vi "lab2_usrp_packet_transceiver2.vi"() -> ()   [LabVIEW 2014]
uses:
  <vilib>/addons/Modulation/Digital/General/MT Generate Bits (Galois, PN Order).vi
  <vilib>/addons/Modulation/Analog/support/mod_Set Error Source.vi
  <vilib>/addons/Modulation/Digital/Support/Common/Validators/mod_Generate Bits Validate.vi
  var_stop.vi
  <vilib>/addons/Modulation/Digital/Support/Common/Validators/mod_Generate Filter Coefficients Validate.vi
  <vilib>/addons/Modulation/Digital/General/subVIs/mod_Generate Filter Coefficients.vi
  <vilib>/measure/maspectr.llb/FFT Power Spectrum and PSD for 1 Chan (CDB).vi
  <vilib>/addons/Modulation/Digital/General/MT Apply Matched Filter (Generic).vi
  <vilib>/addons/Modulation/Digital/General/MT Align to Ideal Symbols (Generic).vi
  <instrlib>/niUSRP/niUSRP Fetch Rx Data (CDB Cluster).vi
  <instrlib>/niUSRP/niUSRP Write Tx Data (CDB Cluster).vi
  <vilib>/addons/Modulation/Digital/General/subVIs/mod_Generate Bits PN Sequence.vi
  <vilib>/addons/Modulation/Digital/General/MT Apply Pulse Shaping Filter (Generic).vi
  <vilib>/addons/Modulation/niDMT.lvlib
  <vilib>/measure/NI_MAPro.lvlib
panel:
  out "ser":dbl
  out "received symbols":dbl
  out "error symbols":i32
  in  "random bits length":i32=50000
  in  "packet bits":i32[](array[numeric])
  out "RX Constellation Map (uneq)":cdb[](graph)
  in  "Transmit power (db)":dbl
  out "ber":dbl
  out "received bits":i32
  out "error bits":i32
  in  "random bits":i8[](array[numeric])
  out "found?":bool
  out "# elements in queue":i32
  out "Spectrum monitor":cluster{"f0":dbl, "df":dbl, "magnitude":dbl[]}(graph)={"f0"=-0.49993781867926873, "df"=0.00012436264146250465, "magnitude"=[]}
  out "RX Constellation Map":cdb[](graph)
  out "valid?":bool
  in  "Gray code?":bool
  in  "Modulation":enum16{"PSK", "QAM"}(ring)=enum."QAM"
  out "Rx String":string
  out "packet len":u32
  in  "Send":bool
  in  "filter length (symbols)":i32=8
  in  "filter parameter":dbl=0.5 format="%.2f"
  in  "pulse shaping filter (none)":T1(ring)=enum."Raised Cosine"
  in  "M-PSK (4)":i32=16 caption="M-ARY"
  in  "samples per symbol (16)":i32=4
  out "packet bits length":i32
  in  "number of samples":i64=40000
  out "RX coerced gain":dbl format="%#_6f"
  out "RX coerced carrier frequency":dbl=915000000.0 format="%#_6p"
  out "RX coerced IQ rate":dbl=4000000.0 format="%#_6p"
  in  "RX active antenna":string="RX2"
  in  "RX gain":dbl format="%#_6f"
  in  "RX device names":refnum<k15>="192.168.10.2"
  out "TX coerced gain":dbl format="%#_6f"
  out "TX coerced carrier frequency":dbl=915000000.0 format="%#_6p"
  out "coerced IQ rate":dbl=4000000.0 format="%#_6p"
  in  "TX device names":refnum<k15>="192.168.10.2"
  in  "TX gain":dbl format="%#_6f"
  in  "carrier frequency":dbl=915000000.0 format="%#_6p"
  in  "IQ rate":dbl=800000.0 format="%#_6p"
  in  "stop":bool
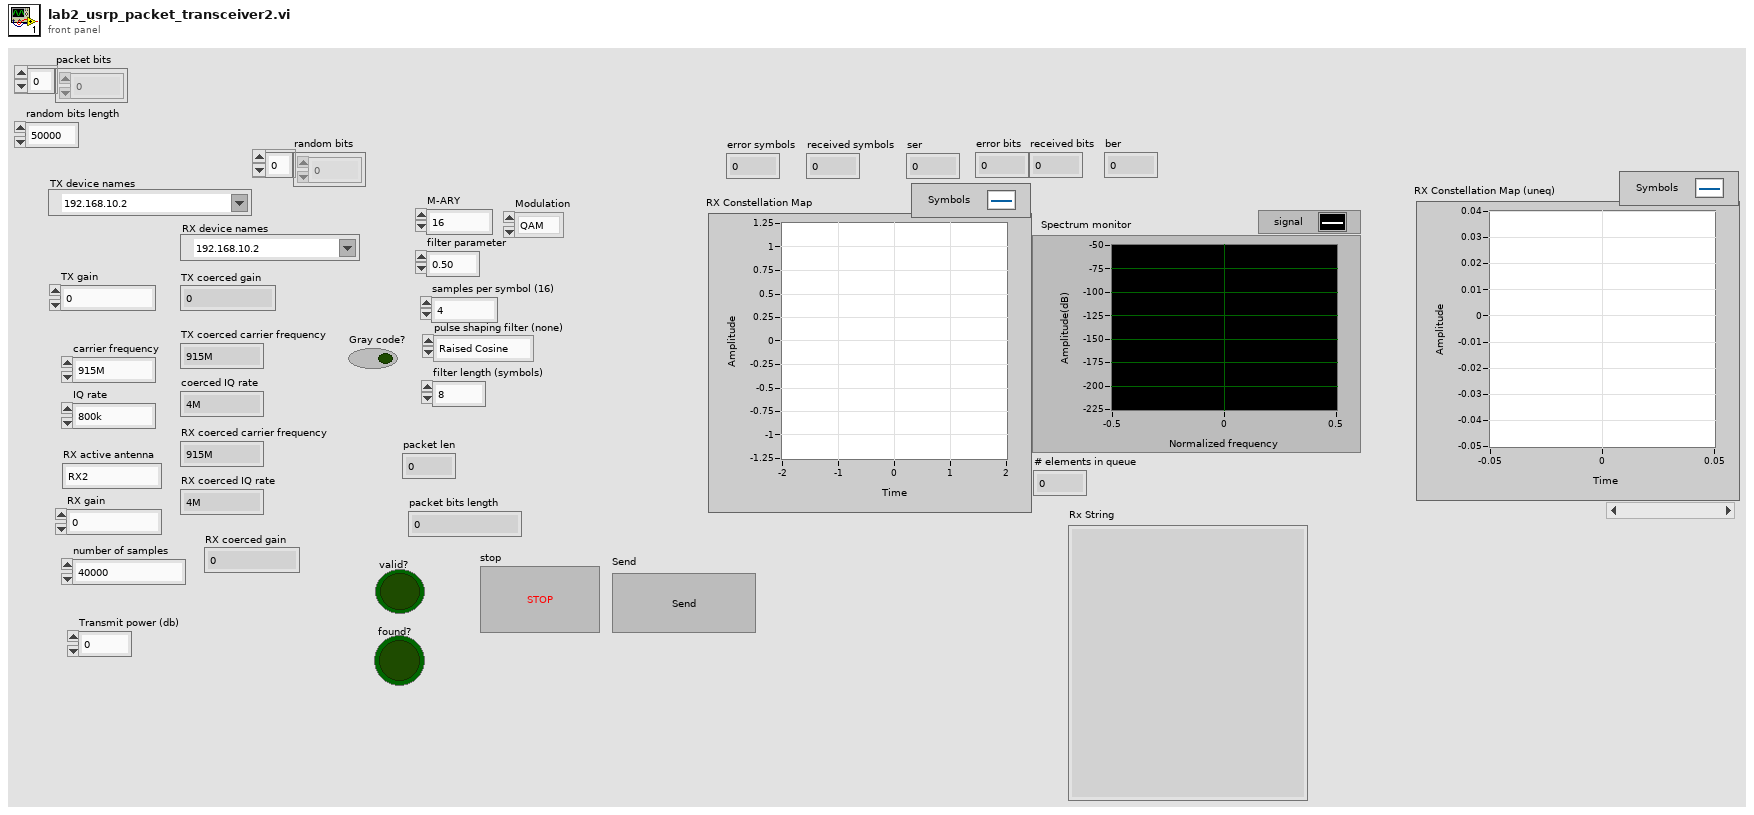
[diagram p1: front panel]
types:
  T1 = enum16{"none", "Raised Cosine", "Root Raised Cos", "Gaussian"}
  T2 = enum16{"FSK", "PSK", "QAM", "MSK", "PAM", "ASK", "CPM"}
  T3 = cluster{"samples per symbol (16)":i32, "symbol map":cdb[], "index map":u32[]}
  T4 = cluster{"samples per symbol (16)":i32, "symbol map":cdb[], i32[]}
  T5 = typedef "niAMT.lvlib/Complex Data Waveform.ctl" = cluster{"t0":dbl, "dt":dbl, "Y":cdb[]}
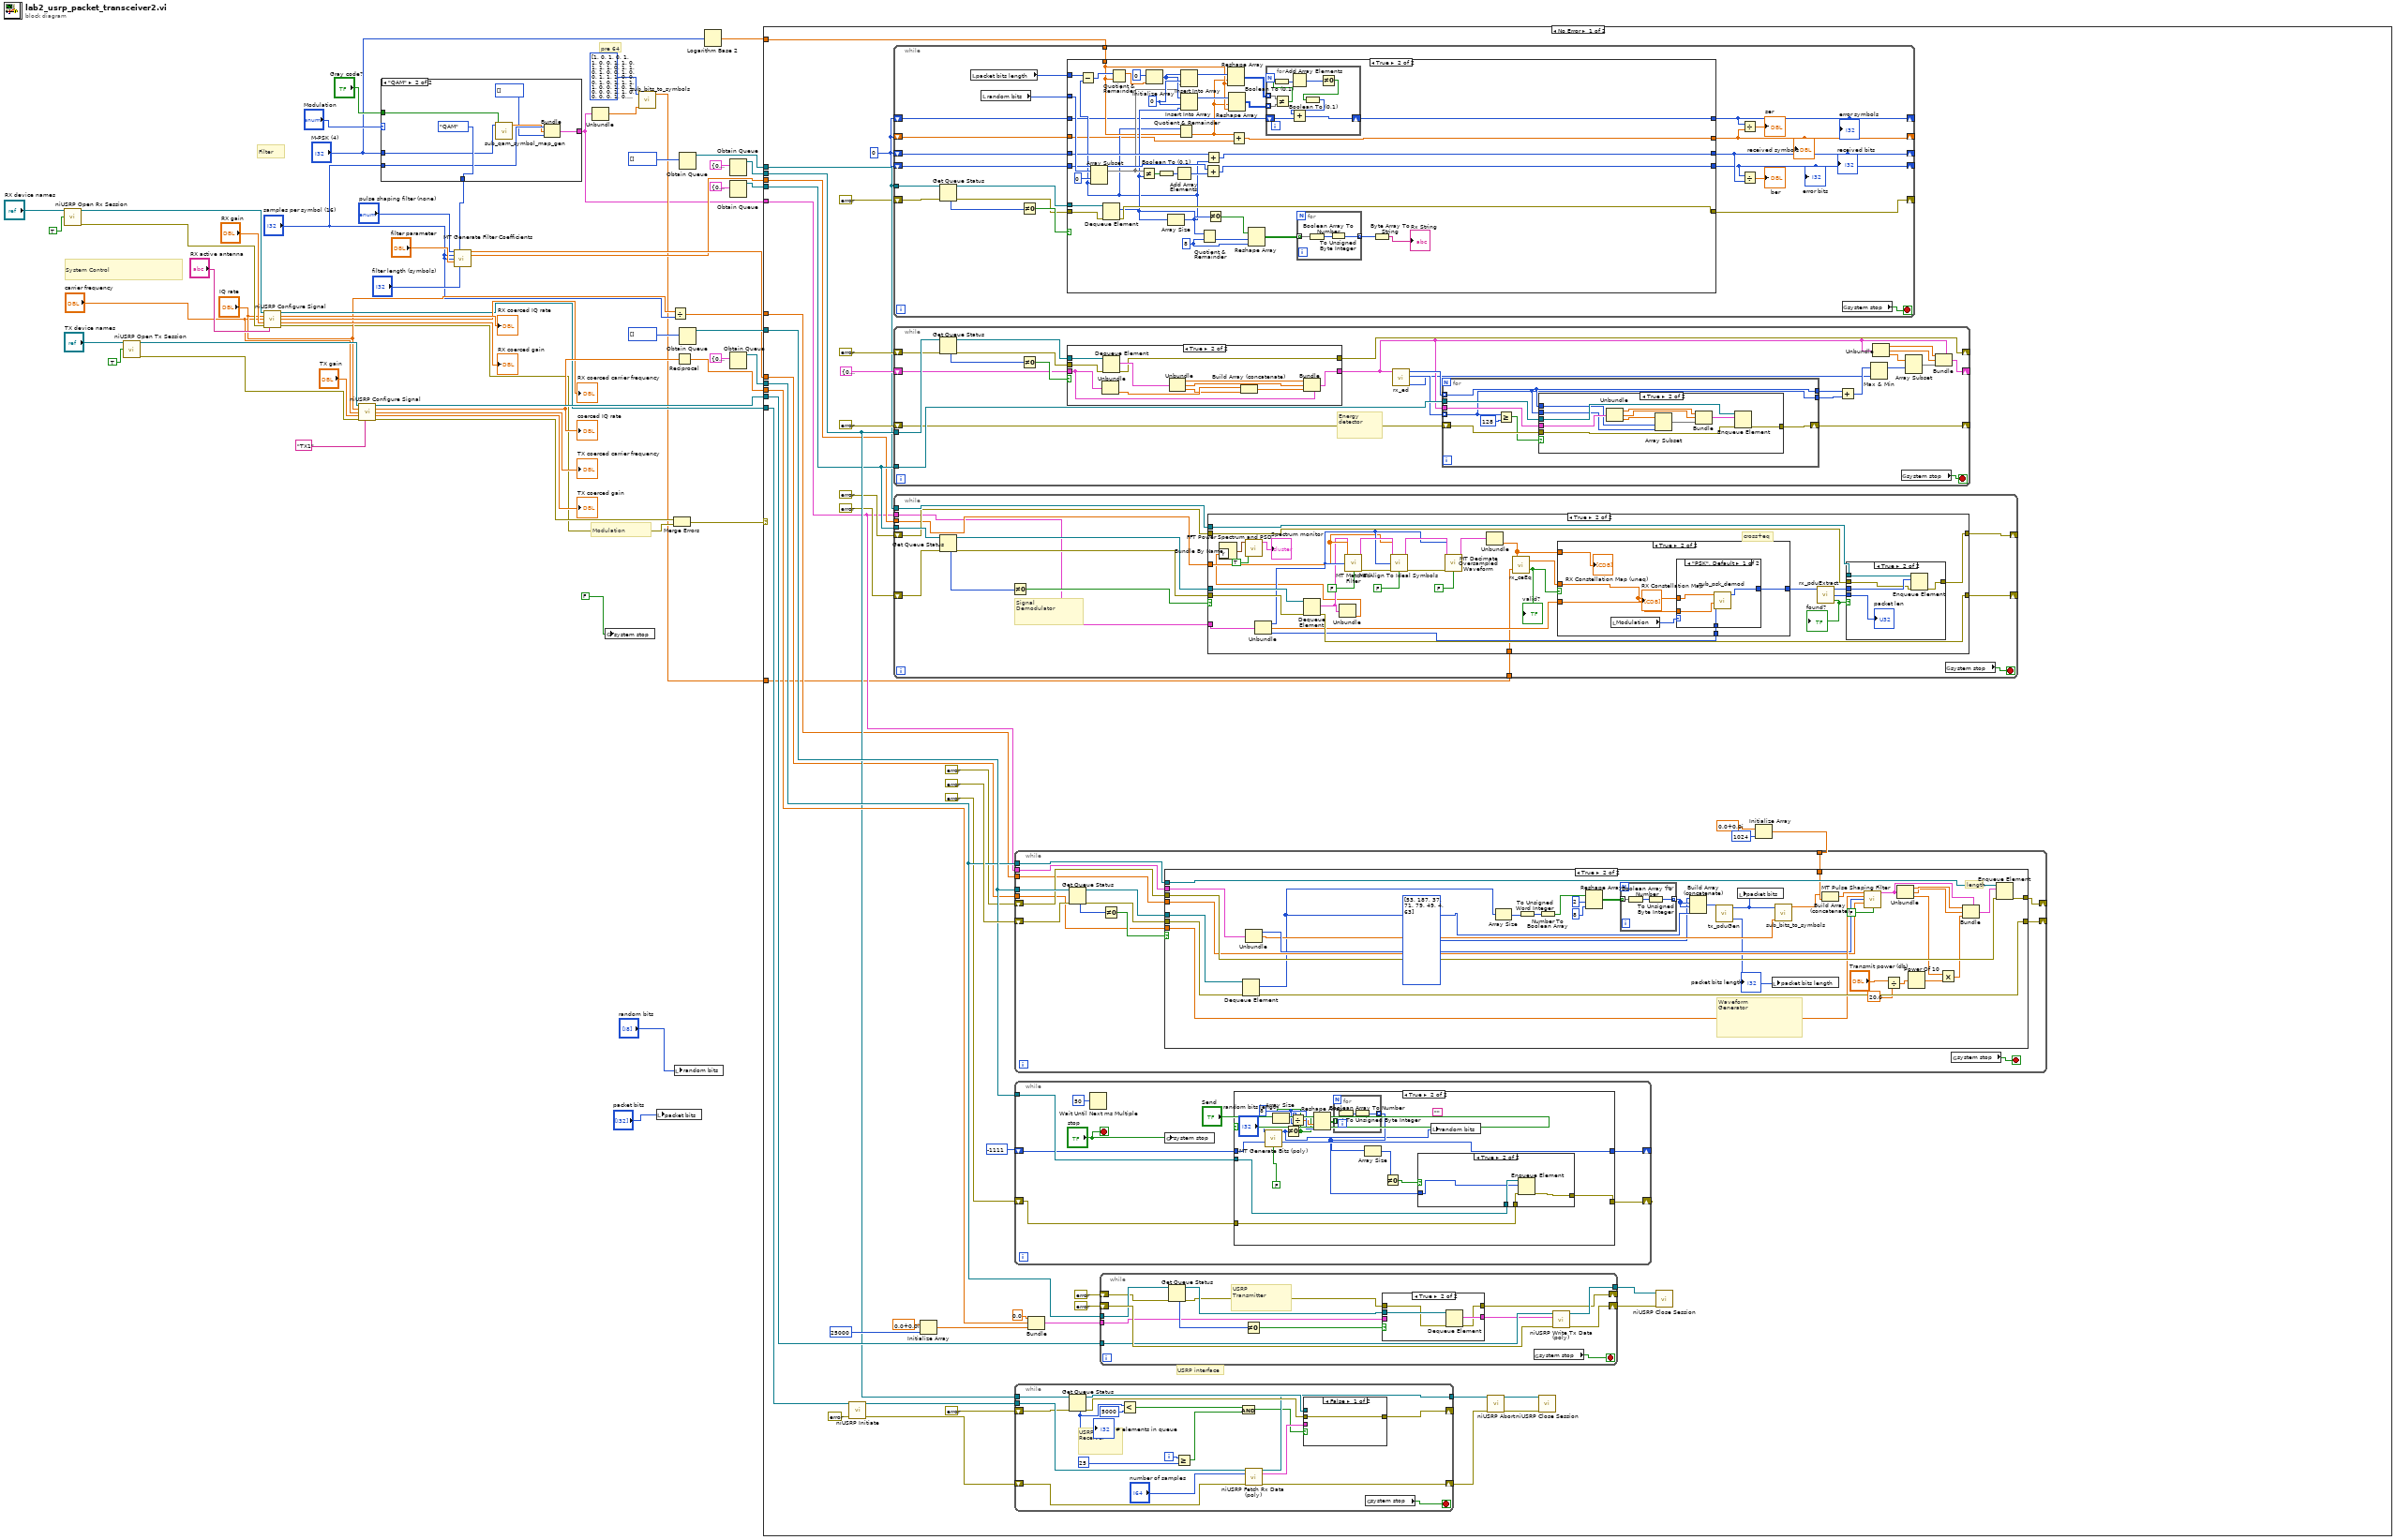
[diagram p0: block diagram]
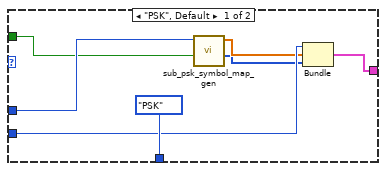
[diagram p2: hidden frame]
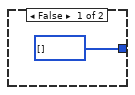
[diagram p5: hidden frame]
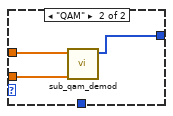
[diagram p6: hidden frame]
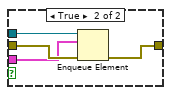
[diagram p10: hidden frame]
diagram:
  # "pre 64"
  # "Modulation"
  # "Filter"
  # "System Control"
  n1 = call <instrlib>:"niUSRP Open Rx Session.vi"("device names"="RX device names", "reset"=TRUE) -> ("session handle out"=w41:refnum<k15>, "error out"=w40:errorcluster)  [unwired: 12 in]
  n2 = call <instrlib>:"niUSRP Open Tx Session.vi"("device names"="TX device names", "reset"=TRUE) -> ("session handle out"=w54:refnum<k15>, "error out"=w53:errorcluster)  [unwired: 12 in]
  n3 = call <instrlib>:"niUSRP Configure Signal.vi"("session handle"=w41, "IQ rate"="IQ rate", "carrier frequency"="carrier frequency", "gain"="RX gain", "error in (no error)"=w40, "active antenna"="RX active antenna") -> ("session handle out"=w32:refnum<k15>, "coerced IQ rate"=→"RX coerced IQ rate":dbl, "coerced carrier frequency"=→"RX coerced carrier frequency":dbl, "coerced gain"=→"RX coerced gain":dbl, "error out"=w16:errorcluster)  [unwired: 5 in]
  n4 = call <instrlib>:"niUSRP Configure Signal.vi"("session handle"=w54, "IQ rate"="IQ rate", "carrier frequency"="carrier frequency", "gain"="TX gain", "error in (no error)"=w53, "active antenna"="TX1") -> ("session handle out"=w45:refnum<k15>, "coerced IQ rate"=w43:dbl, "coerced carrier frequency"=→"TX coerced carrier frequency":dbl, "coerced gain"=→"TX coerced gain":dbl, "error out"=w17:errorcluster)  [unwired: 5 in]
  "coerced IQ rate" <- w43
  n5 = case shown="\"QAM\"" "Modulation" {
    tunnel: [T2."PSK" ("modulation type") T2."QAM" ("modulation type")] -> w11
    tunnel: "M-PSK (4)" -> [w61 w67]
    tunnel: "Gray code?" -> [w60 w68]
    tunnel: "samples per symbol (16)" -> [w59 w66]
    tunnel: [w56 w63] -> w5
    frame "PSK", Default {
      n6 = call "sub_psk_symbol_map_gen.vi"("Gray code?"=w60, "M-PSK"=w61) -> ("index map"=w57:u32[], "symbol map"=w58:cdb[])  [unwired: 8 in]
      n7 = Bundle("samples per symbol (16)"=w59, "symbol map"=w58, "index map"=w57) -> (w56:T3)  [unwired: 1 in]
    }
    frame "QAM" {
      n8 = call "sub_qam_symbol_map_gen.vi"("Gray code?"=w68, "M-QAM"=w67) -> ("symbol map"=w65:cdb[])  [unwired: 9 in]
      n9 = Bundle("samples per symbol (16)"=w66, "symbol map"=w65, i32[] []) -> (w63:T4)  [unwired: 1 in]
    }
  }
  n10 = call <vilib>:"MT Generate Filter Coefficients.vi"("pulse shaping filter (none)"="pulse shaping filter (none)", "modulation type"=w11, "pulse shaping samples per symbol (16)"="samples per symbol (16)", "matched samples per symbol (16)"="samples per symbol (16)", "filter parameter"="filter parameter", "filter length (symbols)"="filter length (symbols)") -> ("pulse shaping filter coefficients"=w22:dbl[], "matched filter coefficients"=w20:dbl[])  [unwired: 7 in, 1 out]
  n11 = Unbundle(w5) -> ("symbol map"=w7:cdb[])  [unwired: 2 out]
  n12 = global write "var_stop.vi" "system stop"(FALSE) -> ()
  n13 = call "sub_bits_to_symbols.vi"("symbol map"=w7, "bits"=i16[] [1, 0, 1, 0, 1, 1, 0, 0, 1, 1, 0, 1, 1, 1, 0, 1, 1, 0, 1, 0, 0, 1, 0, 0, 1, 1, 1, 0, 0, 0, 1, 0, 1, 1, 1, 1, 0, 0, 1, 0, 1, 0, 0, 0, 1, 1, 0, 0, 0, 0, 1, 0, 0, 0, 0, 0, 1, 1, 1, 1, 1, 1, 0, 0] ("preamble(64) 2")) -> ("symbols"=w6:cdb[])  [unwired: 9 in]
  n14 = local write "packet bits"("packet bits") -> ()
  n15 = Divide(x="IQ rate", y="samples per symbol (16)") -> (x/y=w21:dbl)
  n16 = Merge Errors(w17, w16) -> (w15:errorcluster)
  n17 = local write "random bits"("random bits") -> ()
  n18 = Reciprocal(x=w43) -> (1/x=w42:dbl)
  n19 = Obtain Queue(element data type=i8[] [] ("output bit stream")) -> (queue out=w27:refnum<queue>)  [unwired: 4 in, 2 out]
  n20 = Obtain Queue(element data type=i16[] []) -> (queue out=w55:refnum<queue>)  [unwired: 4 in, 2 out]
  n21 = Logarithm Base 2(1:"M-PSK (4)") -> (0:w2:dbl)
  n22 = Obtain Queue(element data type=cluster{"t0":dbl, "dt":dbl, "Y":cdb[]} {"t0"=0.0, "dt"=0.0, "Y"=[]} ("data")) -> (queue out=w31:refnum<queue>)  [unwired: 4 in, 2 out]
  n23 = Obtain Queue(element data type=cluster{"t0":dbl, "dt":dbl, "Y":cdb[]} {"t0"=0.0, "dt"=0.0, "Y"=[]} ("data")) -> (queue out=w28:refnum<queue>)  [unwired: 4 in, 2 out]
  n24 = Obtain Queue(element data type=cluster{"t0":dbl, "dt":dbl, "Y":cdb[]} {"t0"=0.0, "dt"=1.0, "Y"=[]} ("data")) -> (queue out=w46:refnum<queue>)  [unwired: 4 in, 2 out]
  n25 = case shown="No Error" w15 {
    tunnel: w55 -> [w113 _]
    tunnel: w46 -> [w108 _]
    tunnel: w45 -> [w109 _]
    tunnel: w42 -> [w102 _]
    tunnel: w32 -> [w97 _]
    tunnel: w31 -> [w91 _]
    tunnel: w28 -> [w87 _]
    tunnel: w27 -> [w85 _]
    tunnel: w5 -> [w79 _]
    tunnel: w22 -> [w82 _]
    tunnel: w21 -> [w81 _]
    tunnel: w20 -> [w80 _]
    tunnel: w6 -> [w73 _]
    tunnel: w2 -> [w71 _]
    frame No Error {
      w70 = 0
      # "USRP interface"
      n26 = call <instrlib>:"niUSRP Initiate.vi"("session handle"=w97, "error in (no error)"=errorcluster {"status"=FALSE, "code"=0, "source"=""}) -> ("session handle out"=w96:refnum<k15>, "error out"=w95:errorcluster)  [unwired: 12 in]
      n27 = while {
        tunnel: w85 -> [w135]
        shift-right: [w128] -> _
        shift-left: errorcluster {"status"=FALSE, "code"=0, "source"=""} ("error out") -> [w134]
        shift-right: [w123] -> _
        shift-left: w70 -> [w126]
        shift-right: [w124] -> _
        shift-left: w70 -> [w125]
        tunnel: w71 -> [w120]
        shift-right: [w117] -> _
        shift-left: w70 -> [w119]
        shift-right: [w116] -> _
        shift-left: w70 -> [w118]
        stop <- w133 stop-if-true
        n28 = Get Queue Status(queue=w135, error in (no error)=w134) -> (queue out=w130:refnum<queue>, error out=w129:errorcluster, # elements in queue=w132:i32)  [unwired: 1 in, 5 out]
        n29 = local read "packet bits length"() -> (w121:i32)
        n30 = local read "random bits"() -> (w127:i8[])
        n31 = Not Equal To 0?(x=w132) -> (x != 0?=w131:bool)
        n32 = case shown="True" w131 {
          tunnel: w130 -> [_ w177]
          tunnel: w129 -> [w140 w176]
          tunnel: [w140 w171] -> w128
          tunnel: w127 -> [_ w168]
          tunnel: w126 -> [w139 w164]
          tunnel: [w139 w163] -> w123
          tunnel: [w138 w161] -> w124
          tunnel: w125 -> [w138 w162]
          tunnel: w121 -> [_ w153]
          tunnel: w120 -> [_ w149]
          tunnel: w119 -> [w137 w145]
          tunnel: [w137 w144] -> w117
          tunnel: w118 -> [w136 w143]
          tunnel: [w136 w141] -> w116
          frame False {
          }
          frame True {
            w157 = 0
            w174 = 8 ("y")
            n33 = Dequeue Element(queue=w177, error in (no error)=w176) -> (element=w154:i8[], error out=w171:errorcluster)  [unwired: 1 in, 2 out]
            n34 = Array Size(array=w154) -> (size(s)=w148:i32)
            n35 = Subtract(x=w153, y=w148) -> (x-y=w152:i32)
            n36 = Array Subset(array=w168, index=0, length=w148) -> (w155:i8[])
            n37 = Quotient & Remainder(x=w152, y=w149) -> (x-y*floor(x/y)=w158:dbl)  [unwired: 1 out]
            n38 = Not Equal?(x=w155, y=w154) -> (x != y?=w167:bool[])
            n39 = Initialize Array(0, w158) -> (w156:i32[])
            n40 = Boolean To (0,1)(Boolean=w167) -> (0, 1=w166:i16[])
            n41 = Add Array Elements(numeric array=w166) -> (sum=w165:i16)
            n42 = Quotient & Remainder(x=w148, y=w149) -> (floor(x/y)=w142:dbl)  [unwired: 1 out]
            n43 = Insert Into Array(array=w156, index=w157, new element=w155) -> (w151:i32[])
            n44 = Insert Into Array(array=w156, index=w157, new element=w154) -> (w150:i32[])
            n45 = Quotient & Remainder(x=w148, y=w174) -> (floor(x/y)=w173:i32)  [unwired: 1 out]
            n46 = Add(x=w164, y=w165) -> (x+y=w163:i32)
            n47 = Add(x=w162, y=w148) -> (x+y=w161:i32)
            n48 = Not Equal To 0?(x=w154) -> (x != 0?=w175:bool[])
            n49 = Reshape Array(w151, w142, w149) -> (w147:i32[][])
            n50 = Reshape Array(w150, w142, w149) -> (w146:i32[][])
            n51 = Add(x=w142, y=w143) -> (x+y=w141:dbl)
            n52 = Reshape Array(w175, w173, w174) -> (w172:bool[][])
            n53 = for {
              tunnel: w147 -> [w185] mode=indexing
              tunnel: w146 -> [w186] mode=indexing
              shift-right: [w181] -> w144
              shift-left: w145 -> [w180]
              n54 = Not Equal?(x=w185, y=w186) -> (x != y?=w184:bool[])
              n55 = Boolean To (0,1)(Boolean=w184) -> (0, 1=w183:i16[])
              n56 = Add Array Elements(numeric array=w183) -> (sum=w182:i16)
              n57 = Not Equal To 0?(x=w182) -> (x != 0?=w179:bool)
              n58 = Boolean To (0,1)(Boolean=w179) -> (0, 1=w178:i16)
              n59 = Add(x=w178, y=w180) -> (x+y=w181:i32)
            }
            n60 = for {
              tunnel: w172 -> [w189] mode=indexing
              tunnel: [w188] -> w170 mode=indexing
              n61 = Boolean Array To Number(Boolean array=w189) -> (number=w187:u32)
              n62 = To Unsigned Byte Integer(number=w187) -> (unsigned 8bit integer=w188:u8)
            }
            n63 = Byte Array To String(unsigned byte array=w170) -> (string=→"Rx String":string)
          }
        }
        "error bits" <- w123
        "received bits" <- w124
        "error symbols" <- w117
        "received symbols" <- w116
        n64 = Divide(x=w117, y=w116) -> (x/y=→"ser":dbl)
        n65 = Divide(x=w123, y=w124) -> (x/y=→"ber":dbl)
        n66 = global read "var_stop.vi" "system stop"() -> (w133:bool)
      }
      n67 = while {
        tunnel: w91 -> [w282]
        shift-right: [w275] -> _
        shift-left: errorcluster {"status"=FALSE, "code"=0, "source"=""} ("error out") -> [w281]
        shift-right: [w261] -> _
        shift-left: cluster{"t0":dbl, "dt":dbl, "Y":cdb[]} {"t0"=0.0, "dt"=0.0, "Y"=[]} ("data") -> [w276]
        tunnel: w87 -> [w274]
        shift-right: [w273] -> _
        shift-left: errorcluster {"status"=FALSE, "code"=0, "source"=""} ("error out") -> [w272]
        stop <- w271 stop-if-true
        # "Energy\ndetector"
        n68 = Get Queue Status(queue=w282, error in (no error)=w281) -> (queue out=w277:refnum<queue>, error out=w278:errorcluster, # elements in queue=w280:i32)  [unwired: 1 in, 5 out]
        n69 = Not Equal To 0?(x=w280) -> (x != 0?=w279:bool)
        n70 = case shown="True" w279 {
          tunnel: w278 -> [w304 w315]
          tunnel: w277 -> [_ w314]
          tunnel: w276 -> [w303 w309]
          tunnel: [w304 w306] -> w275
          tunnel: [w303 w305] -> w268
          frame False {
          }
          frame True {
            n71 = Unbundle(w309) -> ("Y"=w312:cdb[])  [unwired: 2 out]
            n72 = Dequeue Element(queue=w314, error in (no error)=w315) -> (element=w313:cluster{"t0":dbl, "dt":dbl, "Y":cdb[]}, error out=w306:errorcluster)  [unwired: 1 in, 2 out]
            n73 = Unbundle(w313) -> ("t0"=w308:dbl, "dt"=w307:dbl, "Y"=w311:cdb[])
            n74 = Build Array (concatenate)(w312, w311) -> (w310:cdb[])
            n75 = Bundle(cluster=w309, "t0"=w308, "dt"=w307, "Y"=w310) -> (w305:cluster{"t0":dbl, "dt":dbl, "Y":cdb[]})
          }
        }
        n76 = call "rx_ed.vi"("Wavefrom"=w268) -> ("first pulse"=w258:i32, "length"=w269:i32[], "start index"=w270:i32[])  [unwired: 8 in]
        n77 = for {
          tunnel: w274 -> [w290]
          tunnel: w268 -> [w287]
          shift-right: [w289] -> w273
          shift-left: w272 -> [w288]
          tunnel: w270 -> [w286] mode=indexing
          tunnel: w269 -> [w285] mode=indexing
          tunnel: [w286] -> w264
          tunnel: [w285] -> w263
          n78 = Greater Or Equal?(x=w285, y=128) -> (x >= y?=w283:bool)
          n79 = case shown="True" w283 {
            tunnel: w290 -> [_ w302]
            tunnel: [w291 w301] -> w289
            tunnel: w288 -> [w291 w300]
            tunnel: w287 -> [_ w299]
            tunnel: w286 -> [_ w293]
            tunnel: w285 -> [_ w292]
            frame False {
            }
            frame True {
              n80 = Unbundle(w299) -> ("t0"=w297:dbl, "dt"=w298:dbl, "Y"=w295:cdb[])
              n81 = Array Subset(array=w295, index=w293, length=w292) -> (w294:cdb[])
              n82 = Bundle("t0"=w297, "dt"=w298, w294) -> (w296:cluster{"t0":dbl, "dt":dbl, cdb[]})  [unwired: 1 in]
              n83 = Enqueue Element(queue=w302, element=w296, error in (no error)=w300) -> (error out=w301:errorcluster)  [unwired: 1 in, 2 out]
            }
          }
        }
        n84 = Add(x=w264, y=w263) -> (x+y=w260:i32)
        n85 = Max & Min(x=w260, y=w258) -> (max(x,y)=w259:i32)  [unwired: 1 out]
        n86 = Unbundle(w268) -> ("t0"=w267:dbl, "dt"=w266:dbl, "Y"=w265:cdb[])
        n87 = global read "var_stop.vi" "system stop"() -> (w271:bool)
        n88 = Array Subset(array=w265, index=w259) -> (w262:cdb[])  [unwired: 1 in]
        n89 = Bundle(cluster=w268, "t0"=w267, "dt"=w266, "Y"=w262) -> (w261:cluster{"t0":dbl, "dt":dbl, "Y":cdb[]})
      }
      n90 = while {
        tunnel: w87 -> [w203]
        shift-right: [w197] -> _
        shift-left: errorcluster {"status"=FALSE, "code"=0, "source"=""} ("error out") -> [w202]
        tunnel: w85 -> [w196]
        shift-right: [w195] -> _
        shift-left: errorcluster {"status"=FALSE, "code"=0, "source"=""} ("error out") -> [w194]
        tunnel: w80 -> [w192]
        tunnel: w79 -> [w191]
        tunnel: w73 -> [w190]
        stop <- w193 stop-if-true
        # "Signal \nDemodulator"
        n91 = Get Queue Status(queue=w203, error in (no error)=w202) -> (queue out=w199:refnum<queue>, error out=w198:errorcluster, # elements in queue=w201:i32)  [unwired: 1 in, 5 out]
        n92 = Not Equal To 0?(x=w201) -> (x != 0?=w200:bool)
        n93 = case shown="True" w200 {
          tunnel: w199 -> [_ w236]
          tunnel: w198 -> [w205 w237]
          tunnel: [w205 w235] -> w197
          tunnel: w196 -> [_ w228]
          tunnel: [w204 w227] -> w195
          tunnel: w194 -> [w204 w226]
          tunnel: w192 -> [_ w215]
          tunnel: w191 -> [_ w219]
          tunnel: w190 -> [_ w211]
          frame False {
          }
          frame True {
            # "cross+eq"
            n94 = Unbundle(w219) -> ("samples per symbol (16)"=w218:i32, "symbol map"=w217:cdb[], "index map"=w216:u32[])
            n95 = Dequeue Element(queue=w236, error in (no error)=w237) -> (element=w210:cluster{"t0":dbl, "dt":dbl, "Y":cdb[]}, error out=w235:errorcluster)  [unwired: 1 in, 2 out]
            n96 = Unbundle(w210) -> ("Y"=w209:cdb[])  [unwired: 2 out]
            n97 = Bundle By Name("Y"=w209) -> (w214:waveform(cdb))  [unwired: 1 in]
            n98 = call-poly <vilib>:"FFT Power Spectrum and PSD.vi"("dB On (F)"=TRUE, "time signal"=w214) -> ("Power Spectrum / PSD"=→"Spectrum monitor":cluster{"f0":dbl, "df":dbl, "magnitude":dbl[]})  [unwired: 6 in, 3 out]
            n99 = call-poly <vilib>:"MT Matched Filter.vi"("input complex waveform"=w210, "matched filter coefficients"=w215, "samples per symbol (16)"=w218, "reset? (T)"=FALSE) -> ("output complex waveform"=w234:T5, "error out"=w233:errorcluster)  [unwired: 10 in]
            n100 = call-poly <vilib>:"MT Align To Ideal Symbols.vi"("input complex waveform"=w234, "matched filter coefficients"=w215, "samples per symbol (16)"=w218, "error in (no error)"=w233, "reset? (T)"=FALSE) -> ("output complex waveform"=w231:T5, "error out"=w232:errorcluster)  [unwired: 8 in, 1 out]
            n101 = call <vilib>:"MT Decimate Oversampled Waveform.vi"("input complex waveform"=w231, "decimation factor"=w218, "error in (no error)"=w232, "reset? (T)"=FALSE) -> ("output complex waveform"=w230:T5)  [unwired: 10 in, 1 out]
            n102 = Unbundle(w230) -> ("Y"=w208:cdb[])  [unwired: 2 out]
            n103 = call "rx_ceEq.vi"("preamble"=w211, "symbols"=w208) -> ("valid?"=w224:bool, "eq symbols"=w225:cdb[])
            "valid?" <- w224
            n104 = case shown="True" w224 {
              tunnel: [i8[] [] ("output bit stream") w242] -> w207
              tunnel: w217 -> [_ w243]
              tunnel: w225 -> [_ w240]
              tunnel: w216 -> [_ w241]
              tunnel: w208 -> [_ w239]
              frame False {
              }
              frame True {
                n105 = local read "Modulation"() -> (w244:enum16{"PSK", "QAM"})
                n106 = case shown="\"PSK\", Default" w244 {
                  tunnel: w240 -> [w248 w251]
                  tunnel: w243 -> [w247 w250]
                  tunnel: [w245 w249] -> w242
                  tunnel: w241 -> [w246 _]
                  frame "PSK", Default {
                    n107 = call "sub_psk_demod.vi"("index map"=w246, "symbol map"=w247, "symbol"=w248) -> ("bitstream"=w245:i16[])  [unwired: 8 in]
                  }
                  frame "QAM" {
                    n108 = call "sub_qam_demod.vi"("symbol map"=w250, "symbol"=w251) -> ("bitstream"=w249:i16[])  [unwired: 9 in]
                  }
                }
                "RX Constellation Map" <- w240
                "RX Constellation Map (uneq)" <- w239
              }
            }
            n109 = call "rx_pduExtract.vi"("output bit stream"=w207) -> ("found?"=w229:bool, "packet len"=w223:u32, "ppdu"=w206:i8[])  [unwired: 2 in]
            "found?" <- w229
            n110 = case shown="True" w229 {
              tunnel: w206 -> [_ w255]
              tunnel: w228 -> [_ w257]
              tunnel: [w252 w256] -> w227
              tunnel: w226 -> [w252 w253]
              tunnel: w223 -> [_ w254]
              frame False {
              }
              frame True {
                n111 = Enqueue Element(queue=w257, element=w255, error in (no error)=w253) -> (error out=w256:errorcluster)  [unwired: 1 in, 2 out]
                "packet len" <- w254
              }
            }
          }
        }
        n112 = global read "var_stop.vi" "system stop"() -> (w193:bool)
      }
      n113 = Initialize Array(cdb 0.0+0.0i, 25000 ("dimension size")) -> (w103:cdb[])
      n114 = while {
        tunnel: w113 -> [w422]
        shift-right: [w420] -> _
        shift-left: errorcluster {"status"=FALSE, "code"=0, "source"=""} ("error out") -> [w421]
        shift-right: [w417] -> _
        shift-left: -1111 -> [w418]
        stop <- "stop" stop-if-true
        n115 = Wait Until Next ms Multiple(millisecond multiple=u32 50) -> ()  [unwired: 1 out]
        n116 = global write "var_stop.vi" "system stop"("stop") -> ()
        n117 = case shown="True" "Send" {
          tunnel: w422 -> [_ w441]
          tunnel: w421 -> [w426 w440]
          tunnel: [w426 w439] -> w420
          tunnel: w418 -> [w425 w436]
          tunnel: [w425 w435] -> w417
          frame False {
          }
          frame True {
            w433 = 8
            (unwired) ""
            n118 = call-poly <vilib>:"MT Generate Bits (poly).vi"("total bits (128)"="random bits length", "seed in (0xD6BF7DF2)"=w436, "reset? (T)"=FALSE) -> ("output bit stream"=w427:i8[], "seed out"=w435:i32)  [unwired: 10 in, 1 out]
            n119 = Not Equal To 0?(x=w427) -> (x != 0?=w428:bool[])
            n120 = Array Size(array=w428) -> (size(s)=w432:i32)
            n121 = Divide(x=w432, y=w433) -> (x/y=w431:dbl)
            n122 = Reshape Array(w428, w431, w433) -> (w430:bool[][])
            n123 = for {
              tunnel: w430 -> [w445] mode=indexing
              tunnel: [w443] -> w429 mode=indexing
              n124 = Boolean Array To Number(Boolean array=w445) -> (number=w444:u32)
              n125 = To Unsigned Byte Integer(number=w444) -> (unsigned 8bit integer=w443:u8)
            }
            n126 = Array Size(array=w429) -> (size(s)=w438:i32)
            n127 = Not Equal To 0?(x=w438) -> (x != 0?=w442:bool)
            n128 = case shown="True" w442 {
              tunnel: w429 -> [_ w447]
              tunnel: w441 -> [_ w450]
              tunnel: w440 -> [w446 w449]
              tunnel: [w446 w448] -> w439
              frame False {
              }
              frame True {
                n129 = Enqueue Element(queue=w450, element=w447, error in (no error)=w449) -> (error out=w448:errorcluster)  [unwired: 1 in, 2 out]
              }
            }
            n130 = local write "random bits"(w427) -> ()
          }
        }
      }
      n131 = while {
        tunnel: w96 -> [w334]
        shift-right: [w322] -> w92
        shift-left: w95 -> [w333]
        tunnel: w91 -> [w331]
        shift-right: [w325] -> _
        shift-left: errorcluster {"status"=FALSE, "code"=0, "source"=""} ("error out") -> [w330]
        tunnel: [w323] -> w93
        i -> [w320]
        stop <- w321 stop-if-true
        # "USRP\nReceiver"
        n132 = Get Queue Status(queue=w331, error in (no error)=w330) -> (queue out=w327:refnum<queue>, error out=w326:errorcluster, # elements in queue=w329:i32)  [unwired: 1 in, 5 out]
        "# elements in queue" <- w329
        n133 = Less?(x=w329, y=5000) -> (x < y?=w318:bool)
        n134 = Greater Or Equal?(x=w320, y=25) -> (x >= y?=w317:bool)
        n135 = And(x=w318, y=w317) -> (x .and. y?=w316:bool)
        n136 = call-poly <instrlib>:"niUSRP Fetch Rx Data (poly).vi"("session handle"=w334, "number of samples"="number of samples", "error in (no error)"=w333) -> ("session handle out"=w323:refnum<k15>, "data"=w324:cluster{"t0":dbl, "dt":dbl, "Y":cdb[]}, "error out"=w322:errorcluster)  [unwired: 9 in, 1 out]
        n137 = case shown="False" w316 {
          tunnel: w327 -> [_ w339]
          tunnel: w326 -> [w335 w338]
          tunnel: [w335 w337] -> w325
          tunnel: w324 -> [_ w336]
          frame False {
          }
          frame True {
            n138 = Enqueue Element(queue=w339, element=w336, error in (no error)=w338) -> (error out=w337:errorcluster)  [unwired: 1 in, 2 out]
          }
        }
        n139 = global read "var_stop.vi" "system stop"() -> (w321:bool)
      }
      n140 = Bundle(0.0, w102, w103) -> (w100:cluster{dbl, dbl, cdb[]})  [unwired: 1 in]
      n141 = while {
        shift-right: [w349] -> w112
        shift-left: errorcluster {"status"=FALSE, "code"=0, "source"=""} ("error out") -> [w347]
        tunnel: [w348] -> w111
        tunnel: w109 -> [w346]
        tunnel: w108 -> [w344]
        shift-right: [w342] -> _
        shift-left: errorcluster {"status"=FALSE, "code"=0, "source"=""} ("error out") -> [w343]
        tunnel: w100 -> [w341]
        stop <- w340 stop-if-true
        # "USRP\nTransmitter"
        n142 = Get Queue Status(queue=w344, error in (no error)=w343) -> (queue out=w351:refnum<queue>, error out=w350:errorcluster, # elements in queue=w353:i32)  [unwired: 1 in, 5 out]
        n143 = Not Equal To 0?(x=w353) -> (x != 0?=w352:bool)
        n144 = case shown="True" w352 {
          tunnel: w351 -> [_ w359]
          tunnel: w350 -> [w354 w358]
          tunnel: [w355 w357] -> w345
          tunnel: [w354 w356] -> w342
          tunnel: w341 -> [w355 _]
          frame False {
          }
          frame True {
            n145 = Dequeue Element(queue=w359, error in (no error)=w358) -> (element=w357:cluster{"t0":dbl, "dt":dbl, "Y":cdb[]}, error out=w356:errorcluster)  [unwired: 1 in, 2 out]
          }
        }
        n146 = global read "var_stop.vi" "system stop"() -> (w340:bool)
        n147 = call-poly <instrlib>:"niUSRP Write Tx Data (poly).vi"("session handle"=w346, "data"=w345, "error in (no error)"=w347) -> ("session handle out"=w348:refnum<k15>, "error out"=w349:errorcluster)  [unwired: 11 in]
      }
      n148 = call <instrlib>:"niUSRP Abort.vi"("session handle"=w93, "error in (no error)"=w92) -> ("session handle out"=w99:refnum<k15>, "error out"=w98:errorcluster)  [unwired: 12 in]
      n149 = call <instrlib>:"niUSRP Close Session.vi"("session handle"=w99, "error in (no error)"=w98) -> ()  [unwired: 13 in, 1 out]
      n150 = call <instrlib>:"niUSRP Close Session.vi"("session handle"=w111, "error in (no error)"=w112) -> ()  [unwired: 13 in, 1 out]
      n151 = Initialize Array(cdb 0.0+0.0i, 1024 ("dimension size")) -> (w74:cdb[])
      n152 = while {
        tunnel: w113 -> [w371]
        shift-right: [w368] -> _
        shift-left: errorcluster {"status"=FALSE, "code"=0, "source"=""} ("error out") -> [w374]
        tunnel: w108 -> [w367]
        shift-right: [w366] -> _
        shift-left: errorcluster {"status"=FALSE, "code"=0, "source"=""} ("error out") -> [w365]
        tunnel: w79 -> [w363]
        tunnel: w82 -> [w362]
        tunnel: w81 -> [w361]
        tunnel: w74 -> [w360]
        stop <- w364 stop-if-true
        n153 = Get Queue Status(queue=w371, error in (no error)=w374) -> (queue out=w369:refnum<queue>, error out=w370:errorcluster, # elements in queue=w373:i32)  [unwired: 1 in, 5 out]
        n154 = Not Equal To 0?(x=w373) -> (x != 0?=w372:bool)
        n155 = case shown="True" w372 {
          tunnel: w370 -> [w376 w413]
          tunnel: w369 -> [_ w412]
          tunnel: [w376 w411] -> w368
          tunnel: w367 -> [_ w406]
          tunnel: [w375 w405] -> w366
          tunnel: w365 -> [w375 w404]
          tunnel: w363 -> [_ w402]
          tunnel: w362 -> [_ w401]
          tunnel: w361 -> [_ w400]
          tunnel: w360 -> [_ w390]
          frame False {
          }
          frame True {
            # "length"
            # "Waveform \nGenerator"
            n156 = Dequeue Element(queue=w412, error in (no error)=w413) -> (element=w387:i16[], error out=w411:errorcluster)  [unwired: 1 in, 2 out]
            n157 = Unbundle(w402) -> ("samples per symbol (16)"=w396:i32, "symbol map"=w389:cdb[])  [unwired: 1 out]
            n158 = Array Size(array=w387) -> (size(s)=w398:i32)
            n159 = To Unsigned Word Integer(number=w398) -> (unsigned 16bit integer=w397:u16)
            n160 = Number To Boolean Array(number=w397) -> (Boolean array=w410:bool[])
            n161 = Reshape Array(w410, 2 ("dimension size"), 8 ("dimension size")) -> (w407:bool[][])
            n162 = for {
              tunnel: w407 -> [w416] mode=indexing
              tunnel: [w414] -> w399 mode=indexing
              n163 = Boolean Array To Number(Boolean array=w416) -> (number=w415:u32)
              n164 = To Unsigned Byte Integer(number=w415) -> (unsigned 8bit integer=w414:u8)
            }
            n165 = Build Array (concatenate)(u8[] [53, 187, 37, 71, 79, 49, 4, 63] ("Array 2"), w399, w399, w387) -> (w403:i16[])
            n166 = call "tx_pduGen.vi"("byte array"=w403) -> ("packet bits length"=w377:i32, "pdu"=w379:i32[])  [unwired: 3 in]
            "packet bits length" <- w377
            n167 = local write "packet bits"(w379) -> ()
            n168 = local write "packet bits length"(w377) -> ()
            n169 = call "sub_bits_to_symbols.vi"("symbol map"=w389, "bits"=w379) -> ("symbols"=w388:cdb[])  [unwired: 9 in]
            n170 = Build Array (concatenate)(w388, w390) -> (w385:cdb[])
            n171 = call-poly <vilib>:"MT Pulse Shaping Filter.vi"("symbols"=w385, "pulse shaping filter coefficients"=w401, "samples per symbol (16)"=w396, "symbol rate (Hz)"=w400, "reset? (T)"=FALSE) -> ("output complex waveform"=w395:T5)  [unwired: 9 in, 1 out]
            n172 = Divide(x="Transmit power (db)", y=20.0) -> (x/y=w382:dbl)
            n173 = Unbundle(w395) -> ("t0"=w394:dbl, "dt"=w393:dbl, "Y"=w381:cdb[])
            n174 = Power Of 10(x=w382) -> (10^x=w380:dbl)
            n175 = Multiply(x=w381, y=w380) -> (x*y=w378:cdb[])
            n176 = Bundle(cluster=w395, "t0"=w394, "dt"=w393, "Y"=w378) -> (w392:T5)
            n177 = Enqueue Element(queue=w406, element=w392, error in (no error)=w404) -> (error out=w405:errorcluster)  [unwired: 1 in, 2 out]
          }
        }
        n178 = global read "var_stop.vi" "system stop"() -> (w364:bool)
      }
    }
    frame Error {
    }
  }
